vi "image_build.vi"(8 "colors":u32[](array[numeric]), 9 "Min":dbl, 10 "Max":dbl, 11 "Data":dbl[][](array[numeric])) -> (2 "image data":T1)   [LabVIEW 2013]
uses:
  <vilib>/Analysis/NI_AALPro.lvlib
  <vilib>/picture/picture.llb/imagedata.ctl
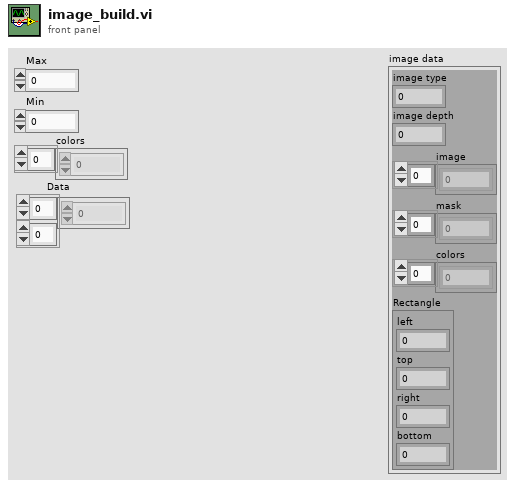
[diagram p1: front panel]
types:
  T1 = typedef "imagedata.ctl" = cluster{"image type":i32, "image depth":i32, "image":u8[], "mask":u8[], "colors":u32[], "Rectangle":cluster{"left":i16, "top":i16, "right":i16, "bottom":i16}}
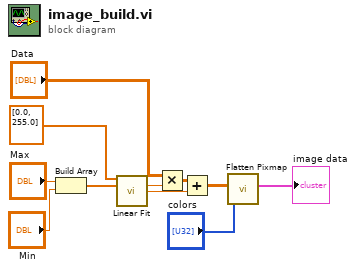
[diagram p0: block diagram]
diagram:
  n1 = Build Array("Max", "Min") -> (w11:dbl[])
  n2 = call <vilib>:"Linear Fit.vi"("Y"=dbl[] [0.0, 255.0], "X"=w11) -> ("slope"=w10:dbl, "intercept"=w8:dbl)  [unwired: 9 in, 3 out]
  n3 = Multiply(x="Data", y=w10) -> (x*y=w9:dbl[][])
  n4 = Add(x=w9, y=w8) -> (x+y=w1:dbl[][])
  n5 = call <vilib>:"Flatten Pixmap.vi"("colors"="colors", "8-bit pixmap"=w1) -> ("image data"=→"image data":T1)  [unwired: 9 in]
